vi "游标显示-油压.vi"(3 "计算参数 in":T1, 5 "reference in":refnum<vi>) -> (0 "计算参数 out":T1, 2 "reference out":refnum<vi>)   [LabVIEW 2013]
panel:
  in  "Array":string[](array[string])=["行程", "油压1"]
  in  "Cursor":T2
  out "Xrange":dbl
  out "Yrange":dbl
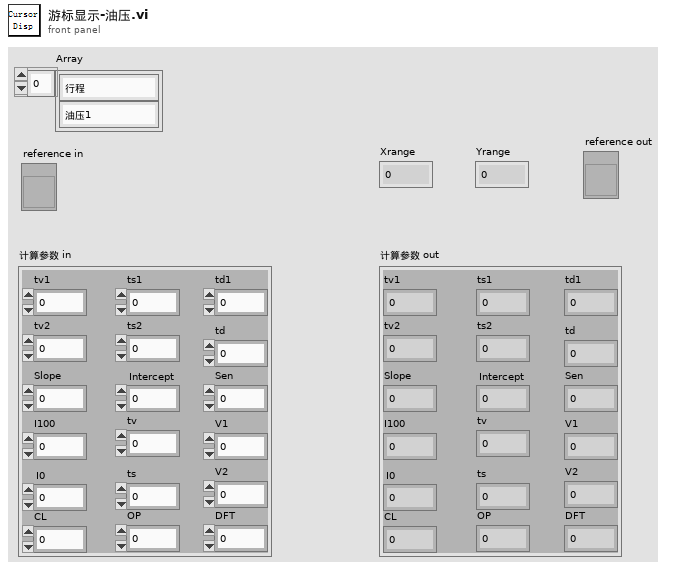
[diagram p1: front panel]
types:
  T1 = cluster{"tv1":dbl, "tv2":dbl, "tv":dbl, "ts1":dbl, "ts2":dbl, "ts":dbl, "td1":dbl, "td":dbl, "Slope":dbl, "Intercept":dbl, "I100":dbl, "I0":dbl, "Sen":dbl, "V1":dbl, "V2":dbl, "CL":dbl, "OP":dbl, "DFT":dbl}
  T2 = cluster{"Name":string, "Color":u32, "Style":u8, "Point Style":u8, "Name Visible":bool, "Allow Drag":bool, "Cursor Mode":u32, "Plot":i32, "Index":i32, "Position":cluster{"X":dbl, "Y":dbl}, "X Scale":u32, "Y Scale":u32, "Watch Plots":i32[], "Watch All Plots":bool, "Plot Area":i32, "Label Offset":cluster{"X":dbl, "Y":dbl}}
  T3 = cluster{"Name":string, "Color":u32, "Style":u8, "Point Style":u8, "Name Visible":bool, "Allow Drag":bool, "Cursor Mode":u32, "Plot":i32, "Index":i32, "Position":cluster{"X":dbl, "Y":dbl}, "X Scale":u32, "Y Scale":u32, "Watch Plots":i32[], "Watch All Plots":bool, "Plot Area":i32, "Label Offset":cluster{"X":dbl, "Y":dbl}}[]
  T4 = typedef "LVCursorListTypeDef.ctl" = cluster{"Name":string, "Color":u32, "Style":u8, "Point Style":u8, "Name Visible":bool, "Allow Drag":bool, "Cursor Mode":u32, "Plot":i32, "Index":i32, "Position":cluster{"X":dbl, "Y":dbl}, "X Scale":u32, "Y Scale":u32, "Watch Plots":i32[], "Watch All Plots":bool, "Plot Area":i32, "Label Offset":cluster{"X":dbl, "Y":dbl}}[]
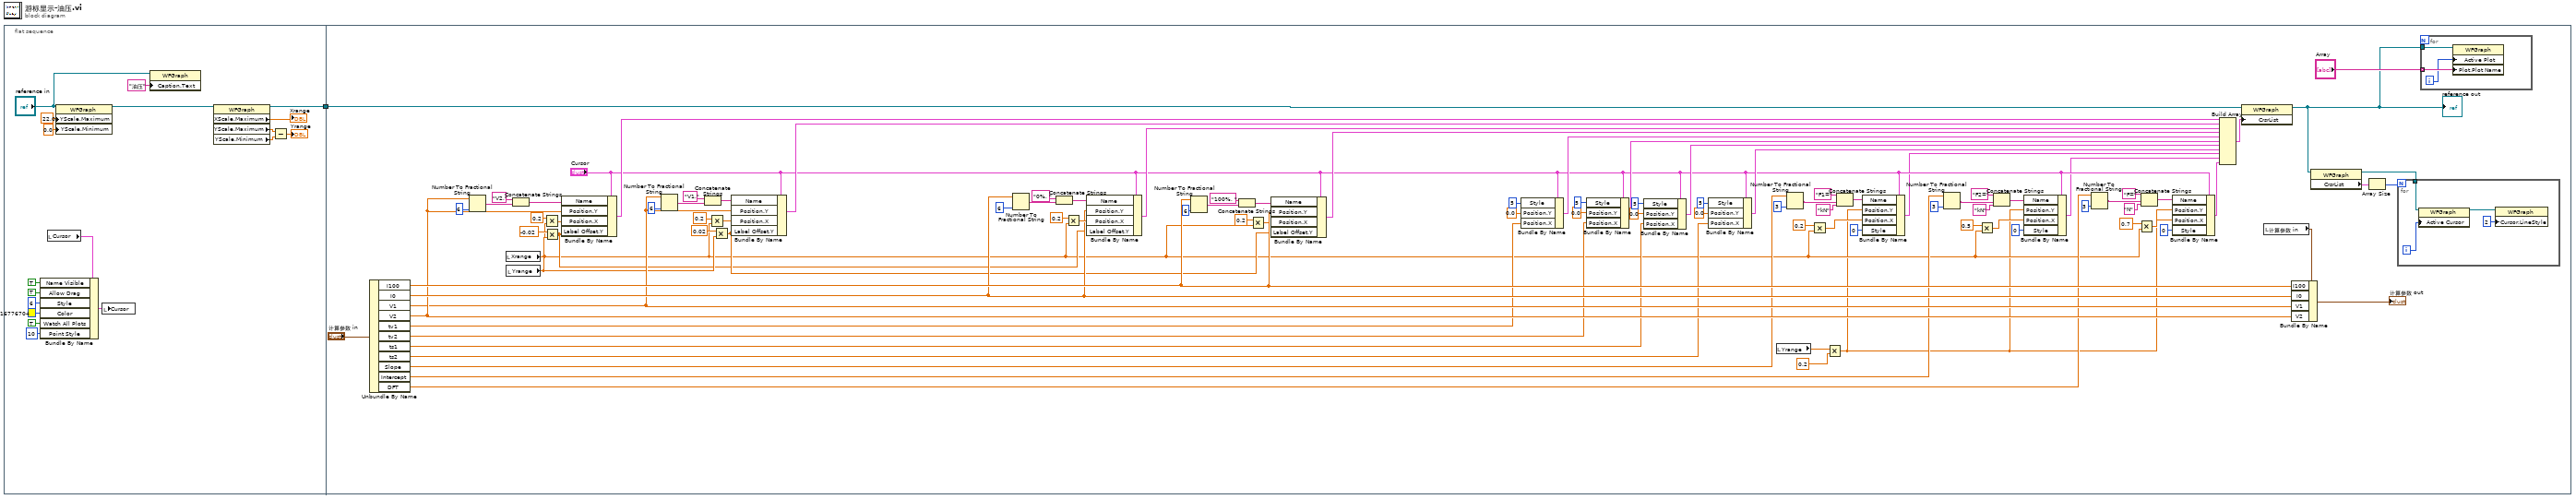
[diagram p0: block diagram]
diagram:
  n1 = flat-sequence {
    tunnel: [w10] -> w1
    tunnel: w1 -> [w83]
    frame #0 {
      n2 = local read "Cursor"() -> (w16:T2)
      n3 = Bundle By Name(cluster=w16, "Name Visible"=TRUE, "Allow Drag"=TRUE, "Style"=u8 6, "Color"=u32 16776704, "Watch All Plots"=TRUE, "Point Style"=u8 10) -> (w15:T2)
      n4 = property on="属性节点" class="WFGraph"(reference="reference in", "YScale.Maximum"=22.0 ("Y标尺.范围:最大值"), "YScale.Minimum"=0.0 ("Y标尺.范围:最小值")) -> (reference out=w2:refnum<vi>)  [unwired: 1 in, 1 out]
      n5 = local write "Cursor"(w15) -> ()
      n6 = property on="Property Node" class="WFGraph"(reference="reference in", "Caption.Text"="油压") -> ()  [unwired: 1 in, 2 out]
      n7 = property class="WFGraph"(reference=w2) -> (reference out=w10:refnum<vi>, "XScale.Maximum"=→"Xrange":dbl, "YScale.Maximum"=w7:dbl, "YScale.Minimum"=w6:dbl)  [unwired: 1 in, 1 out]
      n8 = Subtract(x=w7, y=w6) -> (x-y=→"Yrange":dbl)
    }
    frame #1 {
      n9 = Unbundle By Name("计算参数 in") -> ("I100"=w117:dbl, "I0"=w112:dbl, "V1"=w86:dbl, "V2"=w108:dbl, "tv1"=w78:dbl, "tv2"=w75:dbl, "ts1"=w66:dbl, "ts2"=w65:dbl, "Slope"=w52:dbl, "Intercept"=w33:dbl, "DFT"=w32:dbl)
      n10 = Number To Fractional String(number=w108, precision (6)=i16 6 ("宽度(-)")) -> (F-format string=w92:string)  [unwired: 2 in]
      n11 = local read "Xrange"() -> (w26:dbl)
      n12 = local read "Yrange"() -> (w59:dbl)
      n13 = Concatenate Strings("V2," ("光标.游标名"), w92) -> (w107:string)
      n14 = Multiply(x=0.2 ("y"), y=w26) -> (x*y=w109:dbl)
      n15 = Multiply(x=-0.02, y=w59) -> (x*y=w57:dbl)
      n16 = Bundle By Name(cluster="Cursor", "Name"=w107, "Position.Y"=w108, "Position.X"=w109, "Label Offset.Y"=w57) -> (w103:T2)
      n17 = Number To Fractional String(number=w86, precision (6)=i16 6 ("宽度(-)")) -> (F-format string=w89:string)  [unwired: 2 in]
      n18 = Concatenate Strings("V1," ("光标.游标名"), w89) -> (w87:string)
      n19 = Multiply(x=0.2 ("y"), y=w26) -> (x*y=w85:dbl)
      n20 = Multiply(x=0.02, y=w59) -> (x*y=w58:dbl)
      n21 = Bundle By Name(cluster="Cursor", "Name"=w87, "Position.Y"=w86, "Position.X"=w85, "Label Offset.Y"=w58) -> (w84:T2)
      n22 = Number To Fractional String(number=w112, precision (6)=i16 6 ("宽度(-)")) -> (F-format string=w95:string)  [unwired: 2 in]
      n23 = Concatenate Strings("0%, " ("光标.游标名"), w95) -> (w111:string)
      n24 = Multiply(x=0.2 ("y"), y=w26) -> (x*y=w114:dbl)
      n25 = Bundle By Name(cluster="Cursor", "Name"=w111, "Position.Y"=w112, "Position.X"=w114, "Label Offset.Y"=w57) -> (w104:T2)
      n26 = Number To Fractional String(number=w117, precision (6)=i16 6 ("宽度(-)")) -> (F-format string=w98:string)  [unwired: 2 in]
      n27 = Concatenate Strings("100%, " ("光标.游标名"), w98) -> (w110:string)
      n28 = Multiply(x=0.2 ("y"), y=w26) -> (x*y=w116:dbl)
      n29 = Bundle By Name(cluster="Cursor", "Name"=w110, "Position.Y"=w117, "Position.X"=w116, "Label Offset.Y"=w58) -> (w105:T2)
      n30 = Bundle By Name(cluster="Cursor", "Style"=u8 5, "Position.Y"=0.0, "Position.X"=w78) -> (w70:T2)
      n31 = Bundle By Name(cluster="Cursor", "Style"=u8 5, "Position.Y"=0.0, "Position.X"=w75) -> (w67:T2)
      n32 = Bundle By Name(cluster="Cursor", "Style"=u8 5, "Position.Y"=0.0, "Position.X"=w66) -> (w68:T2)
      n33 = Bundle By Name(cluster="Cursor", "Style"=u8 5, "Position.Y"=0.0, "Position.X"=w65) -> (w69:T2)
      n34 = local read "Yrange"() -> (w23:dbl)
      n35 = Number To Fractional String(number=w52, precision (6)=i16 3 ("宽度(-)")) -> (F-format string=w56:string)  [unwired: 2 in]
      n36 = Multiply(x=0.2, y=w26) -> (x*y=w28:dbl)
      n37 = Multiply(x=w23, y=0.2 ("x")) -> (x*y=w22:dbl)
      n38 = Concatenate Strings("F1=" ("字符串"), w56, "kN" ("字符串")) -> (w51:string)
      n39 = Bundle By Name(cluster="Cursor", "Name"=w51, "Position.Y"=w22, "Position.X"=w28, "Style"=u8 0) -> (w46:T2)
      n40 = Number To Fractional String(number=w33, precision (6)=i16 3 ("宽度(-)")) -> (F-format string=w43:string)  [unwired: 2 in]
      n41 = Multiply(x=0.5, y=w26) -> (x*y=w27:dbl)
      n42 = Concatenate Strings("F2=" ("字符串"), w43, "kN" ("字符串")) -> (w39:string)
      n43 = Bundle By Name(cluster="Cursor", "Name"=w39, "Position.Y"=w22, "Position.X"=w27, "Style"=u8 0) -> (w47:T2)
      n44 = Number To Fractional String(number=w32, precision (6)=i16 3 ("宽度(-)")) -> (F-format string=w38:string)  [unwired: 2 in]
      n45 = Multiply(x=0.7, y=w26) -> (x*y=w25:dbl)
      n46 = Concatenate Strings("F=" ("字符串"), w38, "N" ("字符串")) -> (w34:string)
      n47 = Bundle By Name(cluster="Cursor", "Name"=w34, "Position.Y"=w22, "Position.X"=w25, "Style"=u8 0) -> (w48:T2)
      n48 = Build Array(w103, w84, w104, w105, w70, w67, w68, w69, w46, w47, w48) -> (w106:T3)
      n49 = property class="WFGraph"(reference=w83, "CrsrList"=w106) -> (reference out=w20:refnum<vi>)  [unwired: 1 in, 1 out]
      "reference out" <- w20
      n50 = local read "计算参数 in"() -> (w101:T1)
      n51 = Bundle By Name(cluster=w101, "I100"=w117, "I0"=w112, "V1"=w86, "V2"=w108) -> (→"计算参数 out":T1)
      n52 = property class="WFGraph"(reference=w20) -> (reference out=w62:refnum<vi>, "CrsrList"=w64:T4)  [unwired: 1 in, 1 out]
      n53 = Array Size(array=w64) -> (size(s)=w63:i32)
      n54 = for {
        N: w63 -> [_]
        tunnel: w62 -> [w124]
        i -> [w123]
        n55 = property class="WFGraph"(reference=w124, "Active Cursor"=w123) -> (reference out=w122:refnum<vi>)  [unwired: 1 in, 1 out]
        n56 = property class="WFGraph"(reference=w122, "Cursor.LineStyle"=u8 2 ("Cursor.Line Style")) -> ()  [unwired: 1 in, 2 out]
      }
      n57 = for {
        tunnel: "Array" -> [w120] mode=indexing
        tunnel: w20 -> [w119]
        i -> [w118]
        n58 = property class="WFGraph"(reference=w119, "Active Plot"=w118, "Plot.Plot Name"=w120) -> ()  [unwired: 1 in, 2 out]
      }
    }
  }
